vi "Status.Builder.Read.State.vi"(8 "error in (no error)":errorcluster, 11 "Builder Status in":refnum<class "Status.Builder.lvclass">) -> (0 "error out":errorcluster, 2 "state":T1, 3 "Builder Status out":refnum<class "Status.Builder.lvclass">)   [LabVIEW 2016, in "DSF.Engine.lvlib" / "Status.Builder.lvclass"]
uses:
  Status.Builder.lvclass
  Interface/DSF.Engine.Interface.Builder.Command.ctl
  Status.Builder.lvclass/Status.Builder.ctl
  Status.Builder.State.lvclass
  Interface/DSF.Engine.Interface.Builder.lvclass
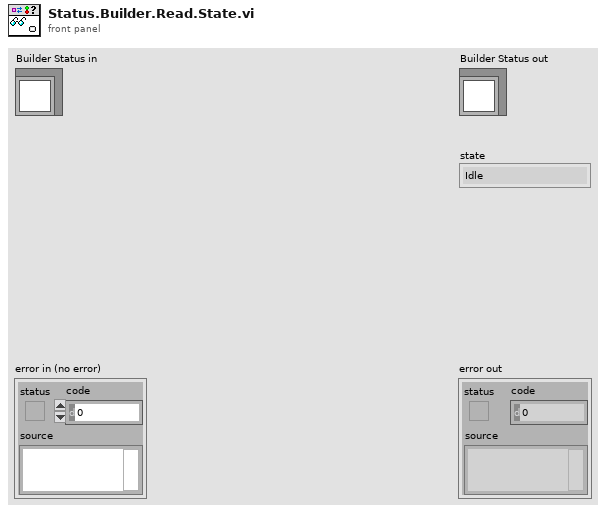
[diagram p1: front panel]
types:
  T1 = typedef "DSF.Engine.lvlib/DSF.Engine.Interface.Builder.lvclass/DSF.Engine.Interface.Builder.Command.ctl" = enum8{"Idle", "Initialize", "Build Buffer", "Parse Buffer", "Shutdown"}
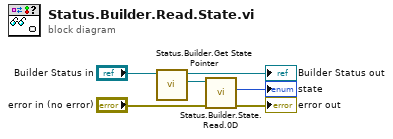
[diagram p0: block diagram]
diagram:
  n1 = call "Status.Builder.Get State Pointer.vi"("Builder Status in"="Builder Status in") -> ("Builder State Pointer"=w5:refnum<class "Status.Builder.State.lvclass">, "Builder Status out"=→"Builder Status out":refnum<class "Status.Builder.lvclass">)  [unwired: 9 in]
  n2 = call "Status.Builder.State.Read.0D.vi"("error in (no error)"="error in (no error)", "Builder State in"=w5) -> ("error out"=→"error out":errorcluster, "state"=→"state":T1)  [unwired: 7 in, 1 out]
